vi "Stop Core.vi"(10 "final error code":i32, 11 "State Pattern in":refnum<class "CoordinatorUI.lvclass">) -> (3 "State Pattern out":refnum<class "CoordinatorUI.lvclass">)   [LabVIEW 2014, in "CoordinatorUI.lvlib" / "CoordinatorUI.lvclass"]
uses:
  CoordinatorUI.lvclass
  CoordinatorUI.lvclass/CoordinatorUI.ctl
  <vilib>/ActorFramework/Stop Msg/Stop Msg.lvclass/Stop Msg.ctl
  <vilib>/ActorFramework/Message Enqueuer/Message Enqueuer.lvclass/Message Enqueuer.ctl
  <vilib>/ActorFramework/Stop Msg/Send Emergency Stop.vi
  <vilib>/ActorFramework/Stop Msg/Send Normal Stop.vi
  <vilib>/ActorFramework/Message Enqueuer/Enqueue Critical.vi
  <vilib>/ActorFramework/Message Enqueuer/Enqueue.vi
  <vilib>/ActorFramework/Message Priority Queue/Priority Enqueue.vi
  Wrapper_lib/zsActor/ActorWrapper.lvclass
  <vilib>/ActorFramework/Stop Msg/Stop Msg.lvclass
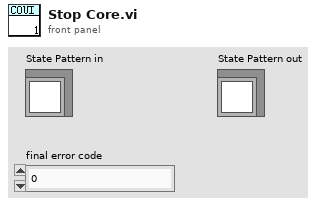
[diagram p1: front panel]
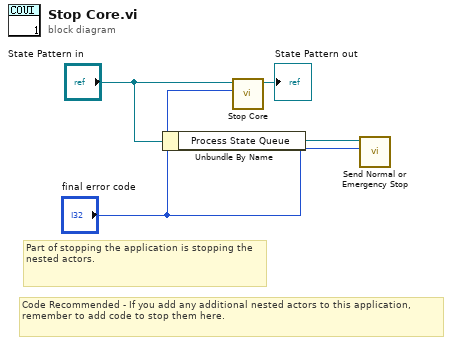
[diagram p0: block diagram]
diagram:
  # "Code Recommended - If you add any additional nested actors to this application, remember to add code to stop them here."
  # "Part of stopping the application is stopping the nested actors."
  n1 = Unbundle By Name("State Pattern in") -> ("Process State Queue"=w2:refnum<class "Message Enqueuer.lvclass">)
  n2 = call-parent "Stop Core.vi"("final error code"="final error code", "Actor in"="State Pattern in") -> ("Actor out"=→"State Pattern out":refnum<class "CoordinatorUI.lvclass">)  [unwired: 9 in]
  n3 = call <vilib>:"Send Normal or Emergency Stop.vi"("final error code"="final error code", "Message Enqueuer"=w2) -> ()  [unwired: 9 in, 1 out]
